vi "SetPgain.vi"(8 "Pgain":dbl, 10 "Controller Channel":i32, 11 "Handle":u32) -> (3 "FT_Status":u32(ring) items=["FT_OK", "FT_INVALID_HANDLE", "FT_DEVICE_NOT_FOUND", "FT_DEVICE_NOT_OPENED", "FT_IO_ERROR", "FT_INSUFFICIENT_RESOURCES", "FT_INVALID_PARAMETER", "FT_INVALID_BAUD_RATE", "FT_DEVICE_NOT_OPENED_FOR_ERASE", "FT_DEVICE_NOT_OPENED_FOR_WRITE", "FT_FAILED_TO_WRITE_DEVICE", "FT_EEPROM_READ_FAILED", "FT_EEPROM_WRITE_FAILED", "FT_EEPROM_ERASE_FAILED", "FT_EEPROM_NOT_PRESENT", "FT_EEPROM_NOT_PROGRAMMED", "FT_INVALID_ARGS", "FT_NOT_SUPPORTED", "FT_OTHER_ERROR"])   [LabVIEW 2011]
panel:
  out "Bytes Written":u32
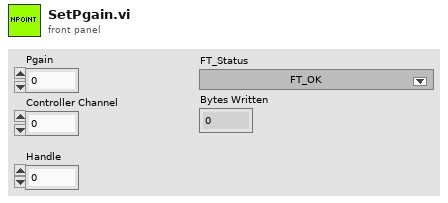
[diagram p1: front panel]
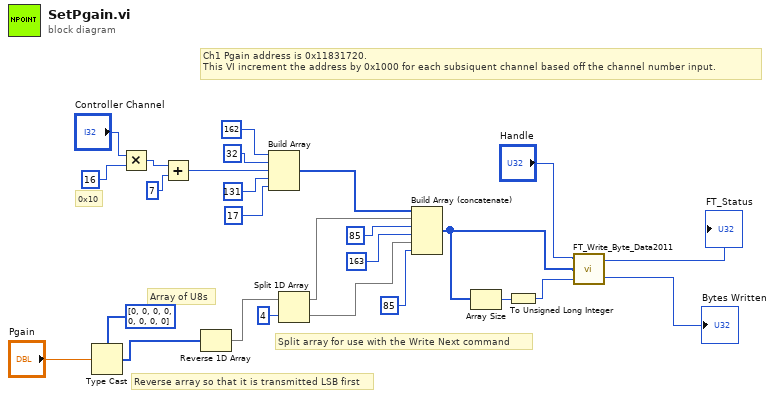
[diagram p0: block diagram]
diagram:
  # "Split array for use with the Write Next command"
  # "Reverse array so that it is transmitted LSB first"
  # "Ch1 Pgain address is 0x11831720.\nThis VI increment the address by 0x1000 for each subsiquent channel based off the channel number input."
  # "0x10"
  # "Array of U8s"
  n1 = Type Cast(type=u8[] [0, 0, 0, 0, 0, 0, 0, 0], x="Pgain") -> (*(type *) &x=w18:u8[])
  n2 = Multiply(x="Controller Channel", y=u8 16) -> (x*y=w14:i32)
  n3 = Add(x=w14, y=7) -> (x+y=w12:i32)
  n4 = Reverse 1D Array(array=w18) -> (reversed array=w11:u8[])
  n5 = Build Array(u8 162 ("element"), u8 32 ("element"), w12, u8 131 ("element"), u8 17 ("element")) -> (w20:i32[])
  n6 = Split 1D Array(array=w11, index=4) -> (first subarray=w9:u8[], second subarray=w6:u8[])
  n7 = Build Array (concatenate)(w20, w9, u8 85 ("element"), u8 163 ("element"), w6, u8 85 ("element")) -> (w4:i32[])
  n8 = Array Size(array=w4) -> (size(s)=w26:i32)
  n9 = To Unsigned Long Integer(number=w26) -> (unsigned 32bit integer=w3:u32)
  n10 = call "FT_Write_Byte_Data2011.vi"("Bytes To Write"=w3, "Buffer"=w4, "Handle"="Handle") -> ("Bytes Written"=→"Bytes Written":u32, "FT_Status"=→"FT_Status":u32)
